vi "SocketWIthKbControll.vi"() -> ()   [LabVIEW 2017]
panel:
  out "Control cluster":T1 {"Roll" scale=-1.0..1.0; "Pitch" scale=-1.0..1.0; "Vertical Speed" scale=-1.0..1.0; "Yaw Speed" scale=-1.0..1.0}
  in  "stop":bool
  out "Python server reply":string
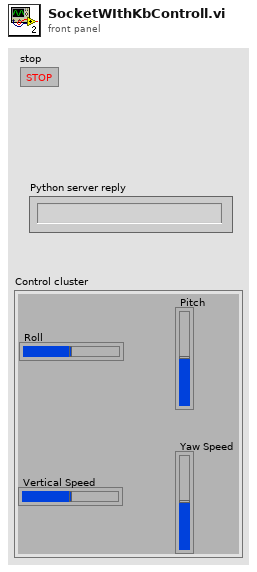
[diagram p1: front panel]
types:
  T1 = cluster{"Roll":dbl, "Pitch":dbl, "Vertical Speed":dbl, "Yaw Speed":dbl}
  T2 = cluster{"Roll":dbl, dbl, "Vertical Speed":dbl, "Yaw Speed":dbl}
  T3 = cluster{dbl, "Pitch":dbl, "Vertical Speed":dbl, "Yaw Speed":dbl}
  T4 = cluster{"Roll":dbl, "Pitch":dbl, dbl, "Yaw Speed":dbl}
  T5 = cluster{"Roll":dbl, "Pitch":dbl, "Vertical Speed":dbl, dbl}
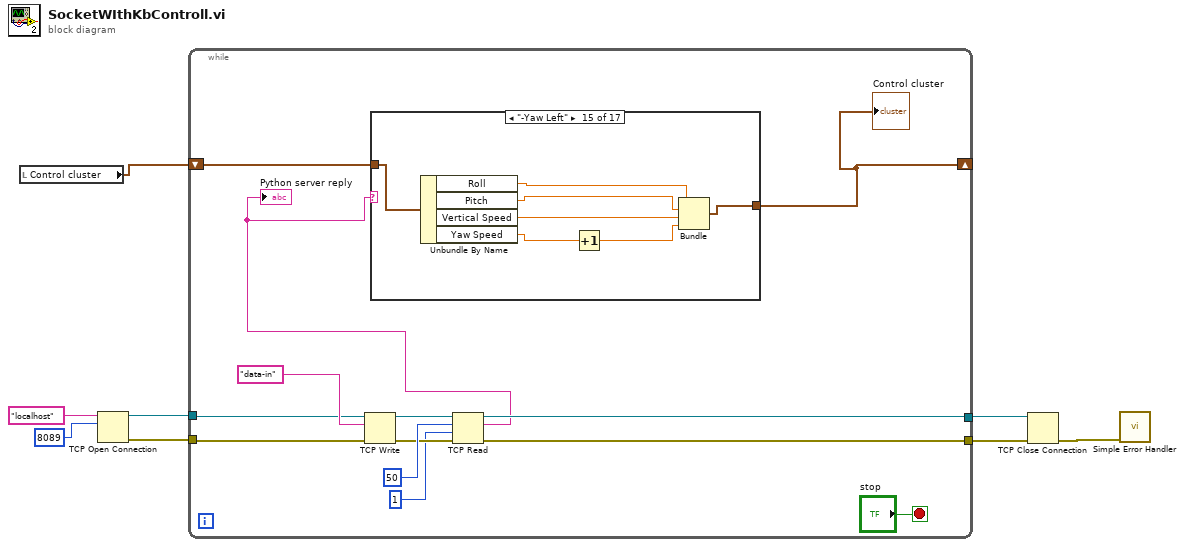
[diagram p0: block diagram]
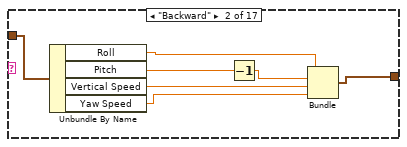
[diagram p3: hidden frame]
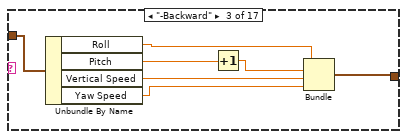
[diagram p4: hidden frame]
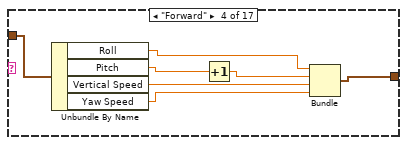
[diagram p5: hidden frame]
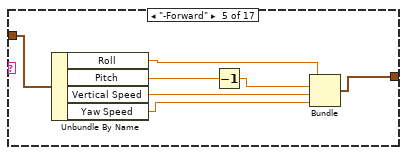
[diagram p6: hidden frame]
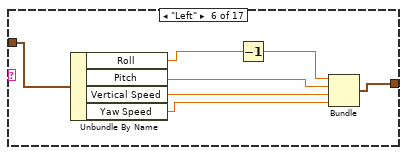
[diagram p7: hidden frame]
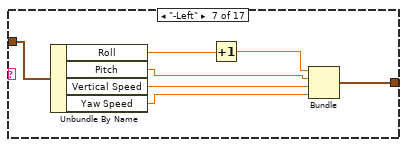
[diagram p8: hidden frame]
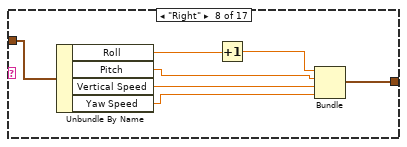
[diagram p9: hidden frame]
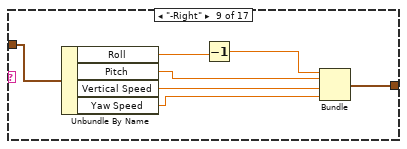
[diagram p10: hidden frame]
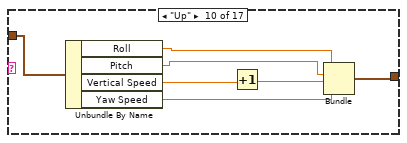
[diagram p11: hidden frame]
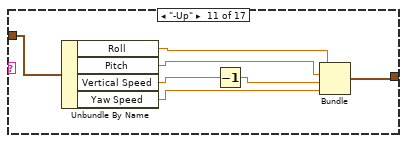
[diagram p12: hidden frame]
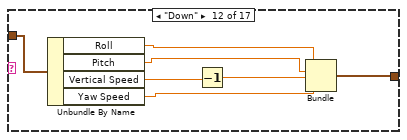
[diagram p13: hidden frame]
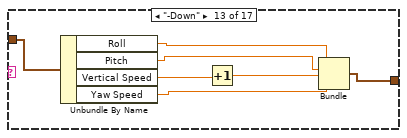
[diagram p14: hidden frame]
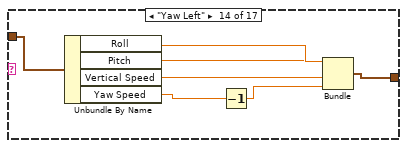
[diagram p15: hidden frame]
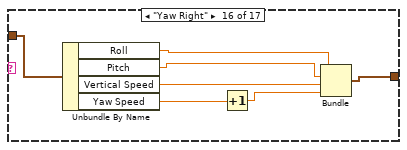
[diagram p16: hidden frame]
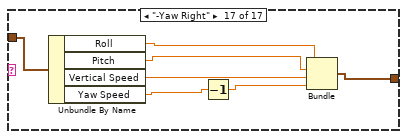
[diagram p17: hidden frame]
diagram:
  n1 = local read "Control cluster"() -> (w1:T1)
  n2 = TCP Open Connection(address="localhost", remote port or service name=u16 8089) -> (connection ID=w2:refnum<k5>, error out=w3:errorcluster)  [unwired: 3 in]
  n3 = while {
    tunnel: [w15] -> w8
    tunnel: [w14] -> w7
    tunnel: w3 -> [w13]
    tunnel: w2 -> [w12]
    shift-right: [w9] -> _
    shift-left: w1 -> [w10]
    stop <- "stop" stop-if-true
    n4 = TCP Write(connection ID=w12, data in="data-in", error in (no error)=w13) -> (connection ID out=w20:refnum<k5>, error out=w19:errorcluster)  [unwired: 1 in, 1 out]
    n5 = TCP Read(connection ID=w20, bytes to read=50, error in (no error)=w19, 9:1 ("timeout ms (25000)")) -> (connection ID out=w15:refnum<k5>, data out=w11:string, error out=w14:errorcluster)  [unwired: 1 in]
    "Python server reply" <- w11
    n6 = case shown="\"-Yaw Left\"" w11 {
      tunnel: [w22 w28 w32 w39 w46 w53 w61 w68 w74 w81 w88 w95 w102 w109 w116 w123 w130] -> w9
      tunnel: w10 -> [w22 w29 w33 w40 w47 w54 w60 w67 w75 w82 w89 w96 w103 w110 w117 w124 w131]
      frame " ", Default {
      }
      frame "Backward" {
        n7 = Unbundle By Name(w29) -> ("Roll"=w27:dbl, "Pitch"=w24:dbl, "Vertical Speed"=w26:dbl, "Yaw Speed"=w25:dbl)
        n8 = Decrement(x=w24) -> (x-1=w23:dbl)
        n9 = Bundle("Roll"=w27, w23, "Vertical Speed"=w26, "Yaw Speed"=w25) -> (w28:T2)  [unwired: 1 in]
      }
      frame "-Backward" {
        n10 = Unbundle By Name(w33) -> ("Roll"=w36:dbl, "Pitch"=w31:dbl, "Vertical Speed"=w35:dbl, "Yaw Speed"=w34:dbl)
        n11 = Increment(x=w31) -> (x+1=w30:dbl)
        n12 = Bundle("Roll"=w36, w30, "Vertical Speed"=w35, "Yaw Speed"=w34) -> (w32:T2)  [unwired: 1 in]
      }
      frame "Forward" {
        n13 = Unbundle By Name(w40) -> ("Roll"=w43:dbl, "Pitch"=w38:dbl, "Vertical Speed"=w42:dbl, "Yaw Speed"=w41:dbl)
        n14 = Increment(x=w38) -> (x+1=w37:dbl)
        n15 = Bundle("Roll"=w43, w37, "Vertical Speed"=w42, "Yaw Speed"=w41) -> (w39:T2)  [unwired: 1 in]
      }
      frame "-Forward" {
        n16 = Unbundle By Name(w47) -> ("Roll"=w50:dbl, "Pitch"=w44:dbl, "Vertical Speed"=w49:dbl, "Yaw Speed"=w48:dbl)
        n17 = Decrement(x=w44) -> (x-1=w45:dbl)
        n18 = Bundle("Roll"=w50, w45, "Vertical Speed"=w49, "Yaw Speed"=w48) -> (w46:T2)  [unwired: 1 in]
      }
      frame "Left" {
        n19 = Unbundle By Name(w54) -> ("Roll"=w52:dbl, "Pitch"=w57:dbl, "Vertical Speed"=w56:dbl, "Yaw Speed"=w55:dbl)
        n20 = Decrement(x=w52) -> (x-1=w51:dbl)
        n21 = Bundle(w51, "Pitch"=w57, "Vertical Speed"=w56, "Yaw Speed"=w55) -> (w53:T3)  [unwired: 1 in]
      }
      frame "-Left" {
        n22 = Unbundle By Name(w60) -> ("Roll"=w59:dbl, "Pitch"=w64:dbl, "Vertical Speed"=w63:dbl, "Yaw Speed"=w62:dbl)
        n23 = Increment(x=w59) -> (x+1=w58:dbl)
        n24 = Bundle(w58, "Pitch"=w64, "Vertical Speed"=w63, "Yaw Speed"=w62) -> (w61:T3)  [unwired: 1 in]
      }
      frame "Right" {
        n25 = Unbundle By Name(w67) -> ("Roll"=w66:dbl, "Pitch"=w71:dbl, "Vertical Speed"=w70:dbl, "Yaw Speed"=w69:dbl)
        n26 = Increment(x=w66) -> (x+1=w65:dbl)
        n27 = Bundle(w65, "Pitch"=w71, "Vertical Speed"=w70, "Yaw Speed"=w69) -> (w68:T3)  [unwired: 1 in]
      }
      frame "-Right" {
        n28 = Unbundle By Name(w75) -> ("Roll"=w73:dbl, "Pitch"=w78:dbl, "Vertical Speed"=w77:dbl, "Yaw Speed"=w76:dbl)
        n29 = Decrement(x=w73) -> (x-1=w72:dbl)
        n30 = Bundle(w72, "Pitch"=w78, "Vertical Speed"=w77, "Yaw Speed"=w76) -> (w74:T3)  [unwired: 1 in]
      }
      frame "Up" {
        n31 = Unbundle By Name(w82) -> ("Roll"=w85:dbl, "Pitch"=w84:dbl, "Vertical Speed"=w80:dbl, "Yaw Speed"=w83:dbl)
        n32 = Increment(x=w80) -> (x+1=w79:dbl)
        n33 = Bundle("Roll"=w85, "Pitch"=w84, w79, "Yaw Speed"=w83) -> (w81:T4)  [unwired: 1 in]
      }
      frame "-Up" {
        n34 = Unbundle By Name(w89) -> ("Roll"=w92:dbl, "Pitch"=w91:dbl, "Vertical Speed"=w87:dbl, "Yaw Speed"=w90:dbl)
        n35 = Decrement(x=w87) -> (x-1=w86:dbl)
        n36 = Bundle("Roll"=w92, "Pitch"=w91, w86, "Yaw Speed"=w90) -> (w88:T4)  [unwired: 1 in]
      }
      frame "Down" {
        n37 = Unbundle By Name(w96) -> ("Roll"=w99:dbl, "Pitch"=w98:dbl, "Vertical Speed"=w94:dbl, "Yaw Speed"=w97:dbl)
        n38 = Decrement(x=w94) -> (x-1=w93:dbl)
        n39 = Bundle("Roll"=w99, "Pitch"=w98, w93, "Yaw Speed"=w97) -> (w95:T4)  [unwired: 1 in]
      }
      frame "-Down" {
        n40 = Unbundle By Name(w103) -> ("Roll"=w106:dbl, "Pitch"=w105:dbl, "Vertical Speed"=w101:dbl, "Yaw Speed"=w104:dbl)
        n41 = Increment(x=w101) -> (x+1=w100:dbl)
        n42 = Bundle("Roll"=w106, "Pitch"=w105, w100, "Yaw Speed"=w104) -> (w102:T4)  [unwired: 1 in]
      }
      frame "Yaw Left" {
        n43 = Unbundle By Name(w110) -> ("Roll"=w113:dbl, "Pitch"=w112:dbl, "Vertical Speed"=w111:dbl, "Yaw Speed"=w108:dbl)
        n44 = Decrement(x=w108) -> (x-1=w107:dbl)
        n45 = Bundle("Roll"=w113, "Pitch"=w112, "Vertical Speed"=w111, w107) -> (w109:T5)  [unwired: 1 in]
      }
      frame "-Yaw Left" {
        n46 = Unbundle By Name(w117) -> ("Roll"=w120:dbl, "Pitch"=w119:dbl, "Vertical Speed"=w118:dbl, "Yaw Speed"=w115:dbl)
        n47 = Increment(x=w115) -> (x+1=w114:dbl)
        n48 = Bundle("Roll"=w120, "Pitch"=w119, "Vertical Speed"=w118, w114) -> (w116:T5)  [unwired: 1 in]
      }
      frame "Yaw Right" {
        n49 = Unbundle By Name(w124) -> ("Roll"=w127:dbl, "Pitch"=w126:dbl, "Vertical Speed"=w125:dbl, "Yaw Speed"=w122:dbl)
        n50 = Increment(x=w122) -> (x+1=w121:dbl)
        n51 = Bundle("Roll"=w127, "Pitch"=w126, "Vertical Speed"=w125, w121) -> (w123:T5)  [unwired: 1 in]
      }
      frame "-Yaw Right" {
        n52 = Unbundle By Name(w131) -> ("Roll"=w134:dbl, "Pitch"=w133:dbl, "Vertical Speed"=w132:dbl, "Yaw Speed"=w129:dbl)
        n53 = Decrement(x=w129) -> (x-1=w128:dbl)
        n54 = Bundle("Roll"=w134, "Pitch"=w133, "Vertical Speed"=w132, w128) -> (w130:T5)  [unwired: 1 in]
      }
    }
    "Control cluster" <- w9
  }
  n55 = TCP Close Connection(connection ID=w8, error in (no error)=w7) -> (error out=w6:errorcluster)  [unwired: 1 in, 1 out]
  n56 = call <vilib>:"Simple Error Handler.vi"("error in (no error)"=w6) -> ()  [unwired: 4 in, 5 out]
